vi "Periodic Tasks.vi"(3 "error in (no error)":errorcluster) -> ()   [LabVIEW 2012]
doc: "This VI runs in parallel to other tasks. It can contain as many user-defined periodic loops as you need. These can carry out PID or other sorts of timed response."
uses:
  <vilib>/Rock Robotics/SystemInterfaces/Utilities/FPGA_UtilitiesLED Source.ctl
  <vilib>/Rock Robotics/SystemInterfaces/Utilities/FPGA_UtilitiesLED State.ctl
  Robot Global Data.vi
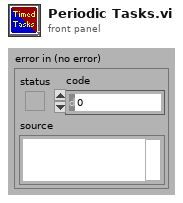
[diagram p1: front panel]
types:
  T1 = typedef "WPI_GyroDevRef.ctl" = cluster{"DevStatus":errorcluster, "Analog Module":T2, "Analog Channel":T3, "Offset":dbl, "Gain (VoltsPerDegree/Second)":dbl}
  T2 = typedef "FPGA_TypedefAnalogModule.ctl" = enum16{"Analog Module 1", "Analog Module 2"}
  T3 = typedef "FPGA_AIChannel.ctl" = enum8{"AI 1", "AI 2", "AI 3", "AI 4", "AI 5", "AI 6", "AI 7", "AI 8", "Invalid"}
  T4 = typedef "WPI_EncoderDevRef.ctl" = cluster{"DevStatus":errorcluster, "EncoderIndex":T5, "CounterIndex":T6, "DistancePerCount":dbl, "Decoding Type":T7}
  T5 = typedef "FPGA_EncoderIdx.ctl" = enum8{"Enc 0", "Enc 1", "Enc 2", "Enc 3", "Invalid"}
  T6 = typedef "FPGA_CounterCtrSystemIndex.ctl" = enum8{"Ctr 0", "Ctr 1", "Ctr 2", "Ctr 3", "Ctr 4", "Ctr 5", "Ctr 6", "Ctr 7", "Invalid"}
  T7 = typedef "WPI_EncoderType.ctl" = enum16{"1x", "2x", "4x"}
  T8 = typedef "FPGA_UtilitiesLED State.ctl" = enum16{"Off", "On", "Toggle"}
  T9 = typedef "FPGA_UtilitiesLED Source.ctl" = enum16{"User LED", "FPGA LED"}
  T10 = typedef "WPI_CompressorDevRef.ctl" = cluster{"DevStatus":errorcluster, "DigitalInputDevRef":T11, "RelayDevRef":T14}
  T11 = typedef "WPI_DigitalInputDevRef.ctl" = cluster{"DevStatus":errorcluster, "DIO Channel":T12, "Digital Module":T13}
  T12 = typedef "FPGA_DIOChannel.ctl" = enum8{"DIO 1", "DIO 2", "DIO 3", "DIO 4", "DIO 5", "DIO 6", "DIO 7", "DIO 8", "DIO 9", "DIO 10", "DIO 11", "DIO 12", "DIO 13", "DIO 14", "Invalid"}
  T13 = typedef "FPGA_TypedefDigitalModule.ctl" = enum16{"Digital Module 1", "Digital Module 2"}
  T14 = typedef "WPI_RelayDevRef.ctl" = cluster{"DevStatus":errorcluster, "Relay Channel":T15, "Digital Module":T13, "Relay Direction":T16}
  T15 = typedef "FPGA_DIORelayChannel.ctl" = enum8{"Relay 1", "Relay 2", "Relay 3", "Relay 4", "Relay 5", "Relay 6", "Relay 7", "Relay 8", "Invalid"}
  T16 = typedef "WPI_RelayDirection.ctl" = enum16{"Both directions", "Forward only", "Reverse only"}
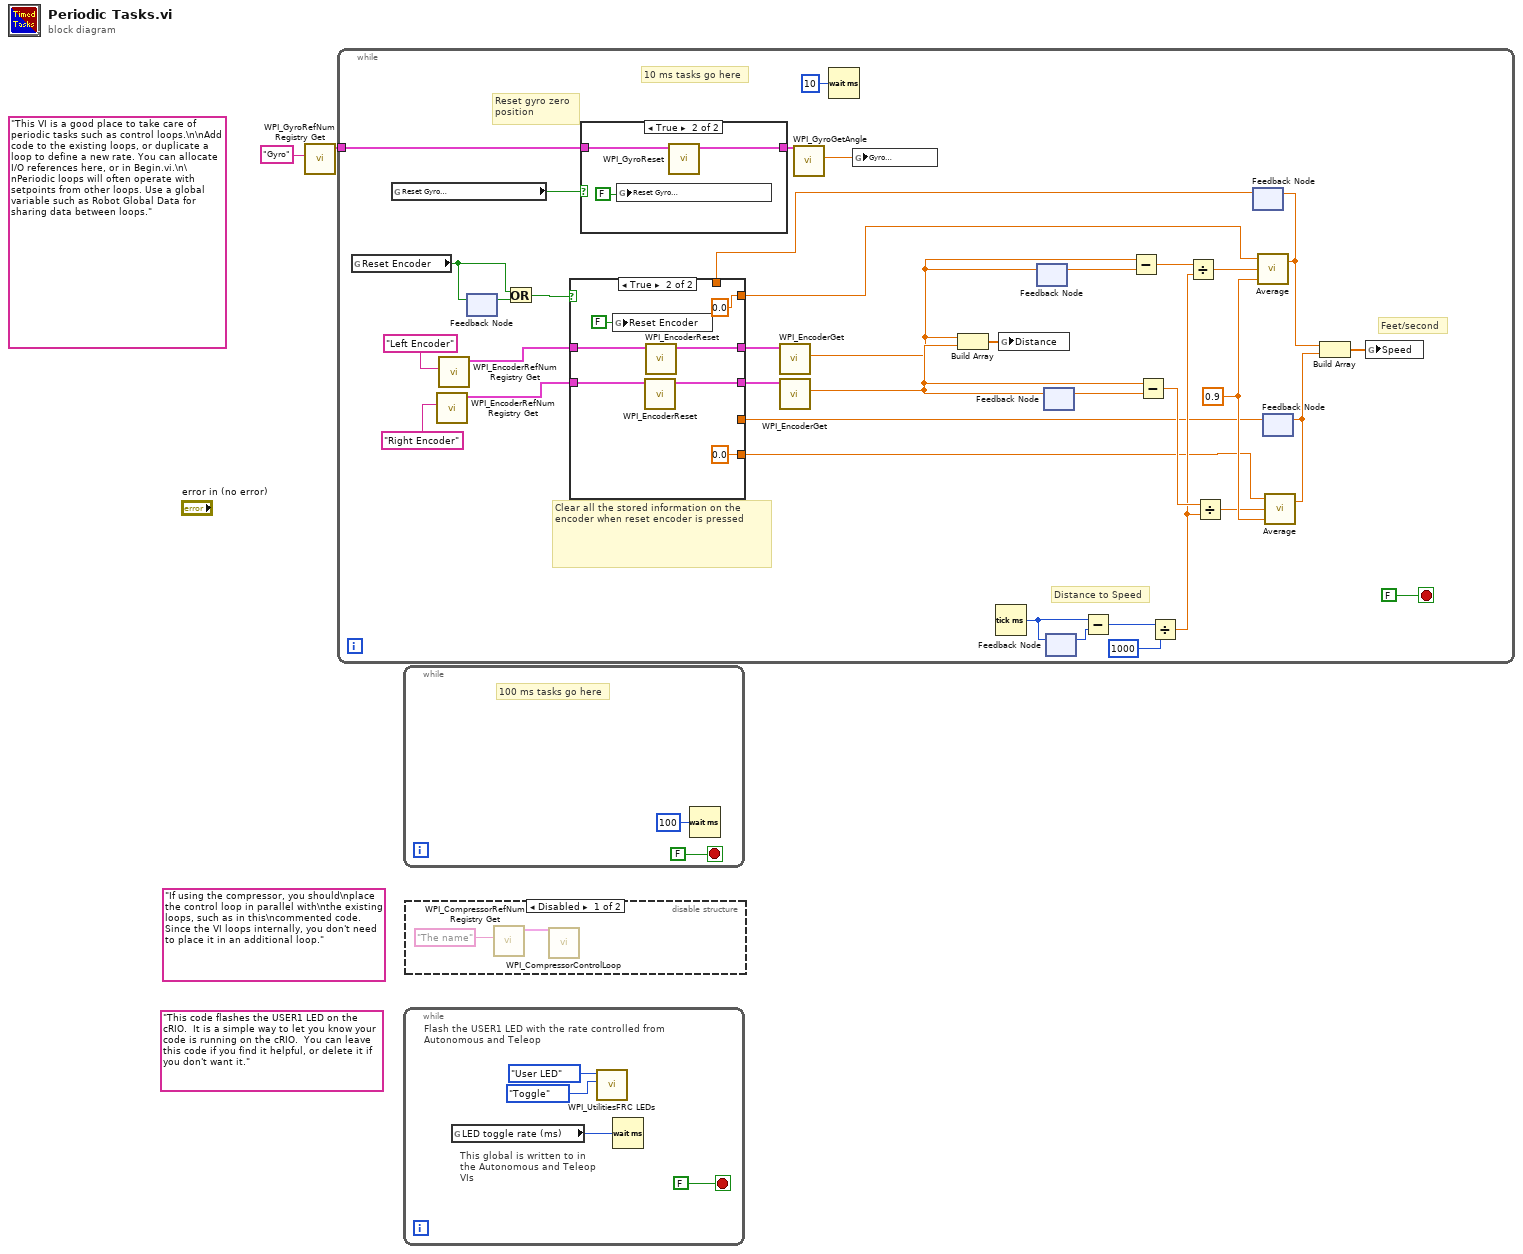
[diagram p0: block diagram]
diagram:
  (unwired) "If using the compressor, you should\nplace the control loop in parallel with\nthe existing loops, such as in this\ncommented code. Since the VI loops internally, you don't need to place it in an additional loop."
  (unwired) "This code flashes the USER1 LED on the cRIO.  It is a simple way to let you know your code is running on the cRIO.  You can leave this code if you find it helpful, or delete it if you don't want it."
  (unwired) "This VI is a good place to take care of periodic tasks such as control loops.\n\nAdd code to the existing loops, or duplicate a loop to define a new rate. You can allocate I/O references here, or in Begin.vi.\n\nPeriodic loops will often operate with setpoints from other loops. Use a global variable such as Robot Global Data for sharing data between loops."
  n1 = call <vilib>:"WPI_GyroRefNum Registry Get.vi"("refnum name"="Gyro") -> ("GyroDevRef"=w2:T1)  [unwired: 9 in, 1 out]
  n2 = while {
    tunnel: w2 -> [w27]
    stop <- FALSE stop-if-true
    w18 = 0.9 ("Speed avg. #")
    # "Reset gyro zero \nposition"
    # "Feet/second"
    # "Distance to Speed"
    # "Clear all the stored information on the encoder when reset encoder is pressed"
    # "10 ms tasks go here"
    n3 = global read "Robot Global Data.vi" "Reset Encoder"() -> (w11:bool)
    n4 = global read "Robot Global Data.vi" "Reset Gyro\nZero Position"() -> (w35:bool)
    n5 = call <vilib>:"WPI_EncoderRefNum Registry Get.vi"("refnum name"="Right Encoder") -> ("EncoderDevRef"=w29:T4)  [unwired: 9 in, 1 out]
    n6 = call <vilib>:"WPI_EncoderRefNum Registry Get.vi"("refnum name"="Left Encoder") -> ("EncoderDevRef"=w32:T4)  [unwired: 9 in, 1 out]
    n7 = feedback-in #1(w11) -> ()
    n8 = feedback #1() -> (w12:bool)  [unwired: 1 in]
    n9 = Or(x=w11, y=w12) -> (x .or. y?=w13:bool)
    n10 = case shown="True" w35 {
      tunnel: w27 -> [w51 w54]
      tunnel: [w51 w53] -> w37
      frame False {
      }
      frame True {
        n11 = global write "Robot Global Data.vi" "Reset Gyro\nZero Position"(FALSE) -> ()
        n12 = call <vilib>:"WPI_GyroReset.vi"("GyroDevRef"=w54) -> ("GyroDevRef"=w53:T1)  [unwired: 10 out]
      }
    }
    n13 = call <vilib>:"WPI_GyroGetAngle.vi"("GyroDevRef"=w37) -> ("Angle"=w36:dbl)  [unwired: 1 in, 9 out]
    n14 = Wait (ms)(milliseconds to wait=u32 10) -> ()  [unwired: 1 out]
    n15 = global write "Robot Global Data.vi" "Gyro\nAngle"(w36) -> ()
    n16 = Tick Count (ms)() -> (millisecond timer value=w25:u32)
    n17 = feedback #2() -> (w24:dbl)  [unwired: 1 in]
    n18 = feedback #3() -> (w19:dbl)  [unwired: 1 in]
    n19 = feedback #4() -> (w26:u32)  [unwired: 1 in]
    n20 = feedback-in #4(w25) -> ()
    n21 = Subtract(x=w25, y=w26) -> (x-y=w22:u32)
    n22 = Divide(x=w22, y=u32 1000) -> (x/y=w17:dbl)
    n23 = feedback #5() -> (w4:dbl)  [unwired: 1 in]
    n24 = feedback #6() -> (w6:dbl)  [unwired: 1 in]
    n25 = case shown="True" w13 {
      tunnel: w32 -> [w43 w50]
      tunnel: [w43 w49] -> w34
      tunnel: w29 -> [w42 w48]
      tunnel: [w42 w47] -> w33
      tunnel: w4 -> [w41 _]
      tunnel: [w41 0.0 ("Output")] -> w3
      tunnel: w6 -> [w40 _]
      tunnel: [w40 0.0 ("Output")] -> w5
      frame False {
      }
      frame True {
        n26 = global write "Robot Global Data.vi" "Reset Encoder"(FALSE ("Reset Encoder")) -> ()
        n27 = call <vilib>:"WPI_EncoderReset.vi"("EncoderDevRef"=w48) -> ("EncoderDevRef"=w47:T4)  [unwired: 1 in, 9 out]
        n28 = call <vilib>:"WPI_EncoderReset.vi"("EncoderDevRef"=w50) -> ("EncoderDevRef"=w49:T4)  [unwired: 1 in, 9 out]
      }
    }
    n29 = call <vilib>:"WPI_EncoderGet.vi"("EncoderDevRef"=w34) -> ("Distance"=w14:dbl)  [unwired: 1 in, 9 out]
    n30 = call <vilib>:"WPI_EncoderGet.vi"("EncoderDevRef"=w33) -> ("Distance"=w16:dbl)  [unwired: 1 in, 9 out]
    n31 = Build Array(w14, w16) -> (w28:dbl[])
    n32 = global write "Robot Global Data.vi" "Distance"(w28) -> ()
    n33 = feedback-in #2(w14) -> ()
    n34 = feedback-in #3(w16) -> ()
    n35 = Subtract(x=w14, y=w24) -> (x-y=w23:dbl)
    n36 = Subtract(x=w16, y=w19) -> (x-y=w20:dbl)
    n37 = Divide(x=w23, y=w17) -> (x/y=w10:dbl)
    n38 = Divide(x=w20, y=w17) -> (x/y=w8:dbl)
    n39 = call "Average.vi"("averg #"=w18, "Input"=w10, "Previous\nValue"=w3) -> ("Output"=w9:dbl)  [unwired: 1 in]
    n40 = feedback-in #5(w9) -> ()
    n41 = call "Average.vi"("averg #"=w18, "Input"=w8, "Previous\nValue"=w5) -> ("Output"=w7:dbl)  [unwired: 1 in]
    n42 = feedback-in #6(w7) -> ()
    n43 = Build Array(w9, w7) -> (w15:dbl[])
    n44 = global write "Robot Global Data.vi" "Speed"(w15) -> ()
  }
  n45 = while {
    stop <- FALSE stop-if-true
    # "100 ms tasks go here"
    n46 = Wait (ms)(milliseconds to wait=u32 100) -> ()  [unwired: 1 out]
  }
  n47 = while {
    stop <- FALSE stop-if-true
    # "This global is written to in the Autonomous and Teleop VIs"
    # "Flash the USER1 LED with the rate controlled from Autonomous and Teleop"
    n48 = global read "Robot Global Data.vi" "LED toggle rate (ms)"() -> (w57:u32)
    n49 = call <vilib>:"WPI_UtilitiesFRC LEDs.vi"("State"=FPGA_UtilitiesLED_State."Toggle", "LED Type"=FPGA_UtilitiesLED_Source."User LED") -> ()  [unwired: 1 in, 9 out]
    n50 = Wait (ms)(milliseconds to wait=w57) -> ()  [unwired: 1 out]
  }
  n51 = disable-structure shown="Disabled" {
    frame Disabled {
      n52 = call <vilib>:"WPI_CompressorRefNum Registry Get.vi"("refnum name"="The name") -> ("CompressorDevRef"=w62:T10)  [unwired: 9 in, 1 out]
      n53 = call <vilib>:"WPI_CompressorControlLoop.vi"("CompressorDevRef"=w62) -> ()  [unwired: 11 in]
    }
    frame Enabled {
    }
  }
